vi "Do.vi"(8 "error in (no error)":errorcluster, 10 "Actor in":refnum<class "Actor.lvclass">, 11 "Write Config File Msg in":refnum<class "Write Config File Msg.lvclass">) -> (0 "error out":errorcluster, 2 "Actor out":refnum<class "Actor.lvclass">)   [LabVIEW 2018, in "MWWL Verification.lvlib" / "Write Config File Msg.lvclass"]
doc: "This VI delivers the message to the actor by calling the appropriate method(s) on the actor."
uses:
  Write Config File Msg.lvclass
  <vilib>/ActorFramework/Actor/Actor.lvclass
  MWWL Verification/MWWL Verification.lvclass
  C:/Program Files (x86)/National Instruments/LabVIEW 2018/vi.lib/ActorFramework/Actor/Actor.lvclass
  Write Config File Msg.lvclass/Write Config File Msg.ctl
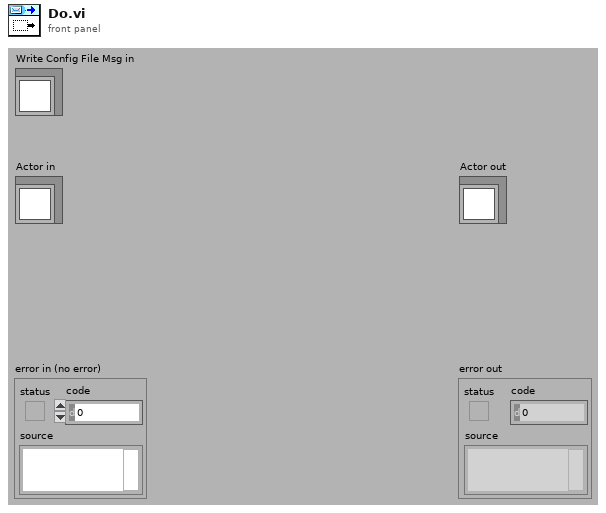
[diagram p1: front panel]
types:
  T1 = typedef "MWWL Verification.lvlib/ConfigSettings.ctl" = cluster{"Base Path":path, "DNL_Configuration Settings.Ports":cluster{"Ref. Range COM Port":refnum<visa-resource-name>, "MWWL COM Port":refnum<visa-resource-name>, "ULS COM Port":refnum<visa-resource-name>, "Laser A COM Port":refnum<visa-resource-name>, "Laser B COM Port":refnum<visa-resource-name>, "Laser C COM Port":refnum<visa-resource-name>, "Laser D COM Port":refnum<visa-resource-name>, "AirMar COM Port":refnum<visa-resource-name>}, "H3611i":bool}
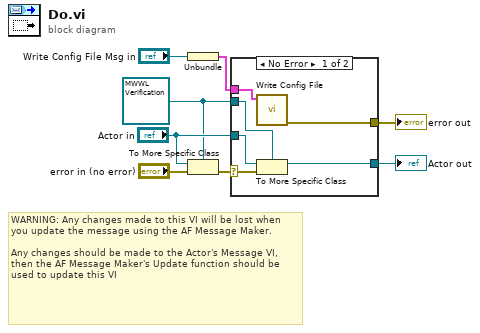
[diagram p0: block diagram]
diagram:
  w3 = refnum<class "MWWL Verification.lvclass"> refnum ("Actor Type")
  # "WARNING: Any changes made to this VI will be lost when you update the message using the AF Message Maker.\n\nAny changes should be made to the Actor's Message VI, then the AF Message Maker's Update function should be used to update this VI"
  n1 = Unbundle("Write Config File Msg in") -> (w2:T1)
  n2 = To More Specific Class(target class=w3, reference="Actor in", error in="error in (no error)") -> (error out=w7:errorcluster)  [unwired: 1 out]
  n3 = case shown="No Error" w7 {
    selector: w7 -> [w14 w16]
    tunnel: [w11 w16] -> w6
    tunnel: [w10 w15] -> w5
    tunnel: "Actor in" -> [w13 w15]
    tunnel: w3 -> [w12 _]
    tunnel: w2 -> [w9 _]
    frame No Error {
      n4 = call "Write Config File.vi"("Settings"=w9) -> ("error out"=w11:errorcluster)  [unwired: 9 in, 1 out]
      n5 = To More Specific Class ("Actor Cast")(target class=w12, reference=w13, error in=w14) -> (specific class reference=w10:refnum<class "MWWL Verification.lvclass">)  [unwired: 1 out]
    }
    frame Error {
    }
  }
  "error out" <- w6
  "Actor out" <- w5
